vi "R1SBRControl.vi"(8 "error constant":errorcluster, 11 "LabVIEW Web Service":refnum<class "Web Service.lvclass">) -> (0 "error out":errorcluster)   [LabVIEW 2016]
uses:
  <vilib>/wsapi/Web Service.lvclass
  R1Controls/R1SBR_SetParams.ctl
  <vilib>/Utility/Variable/NI_VariableUtilities.lvlib
panel:
  out "No phases":i32
  out "current time":timestamp
  out "Numeric":i32
  out "Numeric 2":i32
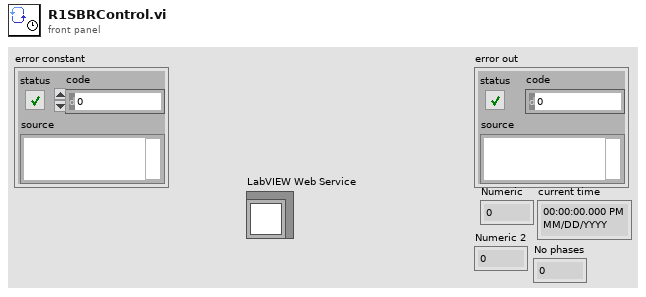
[diagram p1: front panel]
types:
  T1 = cluster{"Media Pump":bool, "Water Pump":bool, "Gas Pump":bool, "Effluent Pump":bool}
  T2 = typedef "R1SBR_SetParams.ctl" = cluster{"Phase":string, "Time, min":dbl, "SBR_Manual":cluster{"Media Pump":bool, "Water Pump":bool, "Gas Pump":bool, "Effluent Pump":bool}}[]
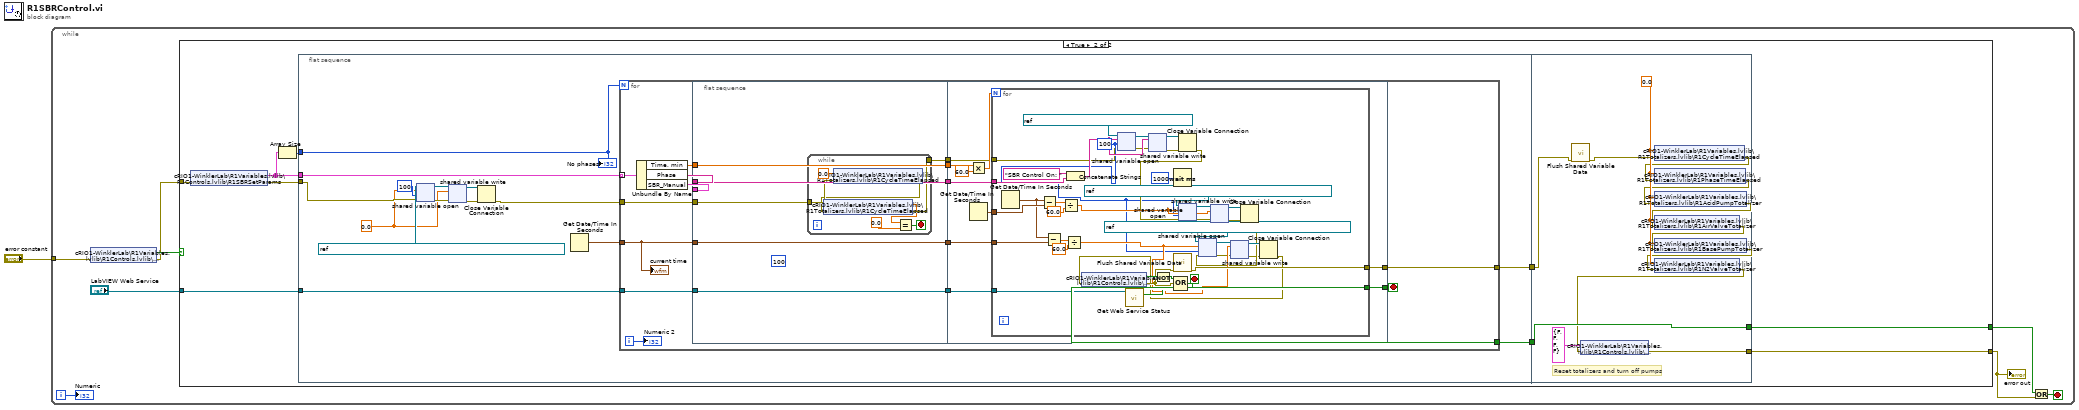
[diagram p0: block diagram]
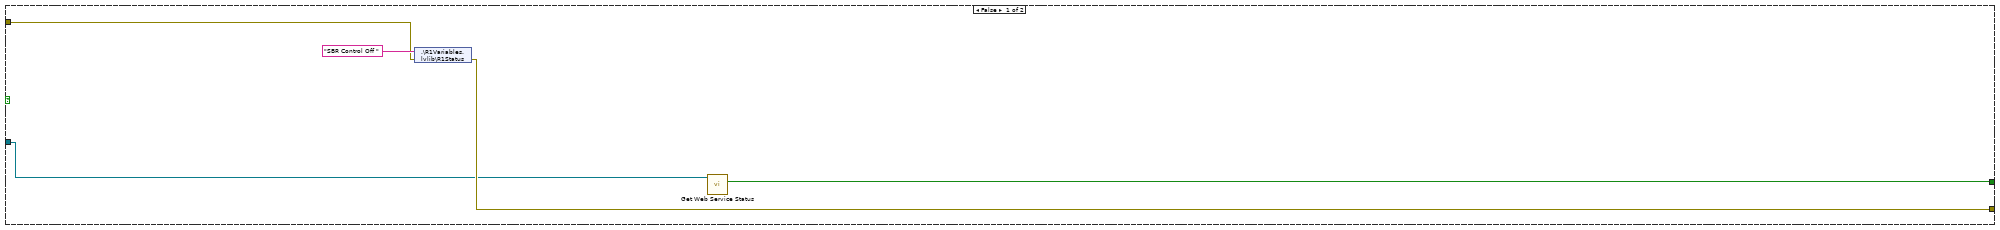
[diagram p2: hidden frame]
diagram:
  n1 = while {
    tunnel: "error constant" -> [w8]
    i -> [w2]
    stop <- w3 stop-if-true
    n2 = shared-variable "cRIO1-WinklerLab\\R1Variables.lvlib\\R1Controls.lvlib\\R1SBRSwitch"(error in=w8) -> (w9:bool, error out=w7:errorcluster)
    n3 = case shown="True" w9 {
      tunnel: "LabVIEW Web Service" -> [w11 w21]
      tunnel: w7 -> [w13 w20]
      tunnel: [w12 w17] -> w5
      tunnel: [w10 w15] -> w4
      frame False {
        n4 = shared-variable ".\\R1Variables.lvlib\\R1Status"("SBR Control Off " ("string"), error in=w13) -> (error out=w12:errorcluster)
        n5 = call <vilib>:"Get Web Service Status.vi"("LabVIEW Web Service"=w11) -> ("service stopping?"=w10:bool)  [unwired: 12 in, 2 out]
      }
      frame True {
        n6 = shared-variable "cRIO1-WinklerLab\\R1Variables.lvlib\\R1Controls.lvlib\\R1SBRSetParams"(error in=w20) -> (w22:T2, error out=w19:errorcluster)
        n7 = Array Size(array=w22) -> (size(s)=w23:i32)
        n8 = flat-sequence {
          tunnel: w22 -> [w37]
          tunnel: w23 -> [w38]
          tunnel: w21 -> [w36]
          tunnel: w19 -> [w26]
          tunnel: [w33] -> w18
          tunnel: [w35] -> w16
          tunnel: w18 -> [w119]
          tunnel: [w121] -> w17
          tunnel: [w120] -> w15
          tunnel: w16 -> [w120]
          frame #0 {
            w24 = 0.0 ("R1CycleTimeElapsed")
            n9 = shared-variable-open(refnum<k21> "ni.var.psp://crio1-winklerlab/R1Variables/R1Totalizers/R1CycleTimeElapsed" ("shared variable refnum in"), w26, w24, 100 ("timeout ms")) -> (w31:refnum<k21>, w29:errorcluster)  [unwired: 2 in]
            n10 = shared-variable-write(w31, w29, w24) -> (w30:refnum<k21>, w28:errorcluster)
            n11 = Close Variable Connection(8:w28, 11:w30) -> (0:w25:errorcluster)
            n12 = Get Date/Time In Seconds() -> (seconds since 1Jan1904=w34:timestamp)
            n13 = for {
              N: w38 -> [_]
              tunnel: w37 -> [w53] mode=indexing
              tunnel: w36 -> [w51]
              tunnel: w25 -> [w45]
              tunnel: [w43] -> w33
              tunnel: [w42] -> w35
              tunnel: w34 -> [w40]
              i -> [w41]
              stop <- w42 stop-if-true
              n14 = Unbundle By Name(w53) -> ("Time, min"=w48:dbl, "Phase"=w47:string, "SBR_Manual"=w52:T1)
              n15 = flat-sequence {
                tunnel: w48 -> [w58]
                tunnel: w52 -> [_]
                tunnel: w51 -> [w59]
                tunnel: [w59] -> w50
                tunnel: [w58] -> w49
                tunnel: w47 -> [w57]
                tunnel: [w57] -> w46
                tunnel: w45 -> [w54]
                tunnel: w40 -> [w56]
                tunnel: [w56] -> w44
                tunnel: [w55] -> w39
                tunnel: [w75] -> w42
                tunnel: w50 -> [w76]
                tunnel: w49 -> [w74]
                tunnel: w46 -> [w71]
                tunnel: w44 -> [w69]
                tunnel: [w68] -> w43
                tunnel: w39 -> [w67]
                frame #0 {
                  (unwired) 100 ("timeout ms")
                  n16 = while {
                    tunnel: w54 -> [w63]
                    tunnel: [w64] -> w55
                    stop <- w65 stop-if-true
                    n17 = shared-variable "cRIO1-WinklerLab\\R1Variables.lvlib\\R1Totalizers.lvlib\\R1CycleTimeElapsed"(0.0 ("R1CycleTimeElapsed"), error in=w63) -> (error out=w61:errorcluster)
                    n18 = shared-variable "cRIO1-WinklerLab\\R1Variables.lvlib\\R1Totalizers.lvlib\\R1CycleTimeElapsed"(error in=w61) -> (w60:dbl, error out=w64:errorcluster)
                    n19 = Equal?(x=w60, y=0.0 ("R1CycleTimeElapsed")) -> (x = y?=w65:bool)
                  }
                }
                frame #1 {
                  n20 = Get Date/Time In Seconds() -> (seconds since 1Jan1904=w70:timestamp)
                  n21 = Multiply(x=w74, y=60.0) -> (x*y=w72:dbl)
                  n22 = for {
                    N: w72 -> [_]
                    tunnel: w76 -> [w105]
                    tunnel: [w114] -> w75
                    tunnel: w71 -> [w112]
                    tunnel: w70 -> [w109]
                    tunnel: w69 -> [w106]
                    tunnel: [w100] -> w68
                    tunnel: w67 -> [w77]
                    stop <- w114 stop-if-true
                    w78 = 100 ("timeout ms")
                    n23 = Get Date/Time In Seconds() -> (seconds since 1Jan1904=w107:timestamp)
                    n24 = Subtract(x=w107, y=w109) -> (x-y=w110:dbl)
                    n25 = Subtract(x=w107, y=w106) -> (x-y=w103:dbl)
                    n26 = Divide(x=w110, y=60.0) -> (x/y=w86:dbl)
                    n27 = Divide(x=w103, y=60.0) -> (x/y=w95:dbl)
                    n28 = Concatenate Strings("SBR Control On: " ("string"), w112) -> (w82:string)
                    n29 = shared-variable-open(refnum<k21> "ni.var.psp://crio1-winklerlab/R1Variables/R1Status" ("shared variable refnum in"), w77, w82, w78) -> (w84:refnum<k21>, w81:errorcluster)  [unwired: 2 in]
                    n30 = call <vilib>:"Get Web Service Status.vi"("LabVIEW Web Service"=w105) -> ("service stopping?"=w104:bool)  [unwired: 12 in, 2 out]
                    n31 = shared-variable-write(w84, w81, w82) -> (w85:refnum<k21>, w80:errorcluster)
                    n32 = Wait (ms)(milliseconds to wait=u32 1000) -> ()  [unwired: 1 out]
                    n33 = Close Variable Connection(8:w80, 11:w85) -> (0:w79:errorcluster)
                    n34 = shared-variable-open(refnum<k21> "ni.var.psp://crio1-winklerlab/R1Variables/R1Totalizers/R1PhaseTimeElapsed" ("shared variable refnum in"), w79, w86, w78) -> (w93:refnum<k21>, w91:errorcluster)  [unwired: 2 in]
                    n35 = shared-variable-write(w93, w91, w86) -> (w94:refnum<k21>, w90:errorcluster)
                    n36 = Close Variable Connection(8:w90, 11:w94) -> (0:w89:errorcluster)
                    n37 = shared-variable-open(refnum<k21> "ni.var.psp://crio1-winklerlab/R1Variables/R1Totalizers/R1CycleTimeElapsed" ("shared variable refnum in"), w89, w95, w78) -> (w98:refnum<k21>, w88:errorcluster)  [unwired: 2 in]
                    n38 = shared-variable-write(w98, w88, w95) -> (w99:refnum<k21>, w87:errorcluster)
                    n39 = Close Variable Connection(8:w87, 11:w99) -> (0:w96:errorcluster)
                    n40 = shared-variable "cRIO1-WinklerLab\\R1Variables.lvlib\\R1Controls.lvlib\\R1SBRSwitch"(error in=w96) -> (w116:bool, error out=w101:errorcluster)
                    n41 = Not(x=w116) -> (.not. x?=w115:bool)
                    n42 = call <vilib>:"Flush Shared Variable Data.vi"("error in (no error)"=w101) -> ("error out"=w100:errorcluster)  [unwired: 10 in]
                    n43 = Compound Arithmetic op=OR(w115, w101, w104) -> (w114:bool)
                  }
                }
              }
              "Numeric 2" <- w41
              "current time" <- w40
            }
            "No phases" <- w38
          }
          frame #1 {
            w127 = 0.0 ("R1CycleTimeElapsed")
            # "Reset totalizers and turn off pumps"
            n44 = call <vilib>:"Flush Shared Variable Data.vi"("error in (no error)"=w119) -> ("error out"=w118:errorcluster)  [unwired: 10 in]
            n45 = shared-variable "cRIO1-WinklerLab\\R1Variables.lvlib\\R1Totalizers.lvlib\\R1CycleTimeElapsed"(w127, error in=w118) -> (error out=w126:errorcluster)
            n46 = shared-variable "cRIO1-WinklerLab\\R1Variables.lvlib\\R1Totalizers.lvlib\\R1PhaseTimeElapsed"(w127, error in=w126) -> (error out=w125:errorcluster)
            n47 = shared-variable "cRIO1-WinklerLab\\R1Variables.lvlib\\R1Totalizers.lvlib\\R1AcidPumpTotalizer"(w127, error in=w125) -> (error out=w124:errorcluster)
            n48 = shared-variable "cRIO1-WinklerLab\\R1Variables.lvlib\\R1Totalizers.lvlib\\R1AirValveTotalizer"(w127, error in=w124) -> (error out=w123:errorcluster)
            n49 = shared-variable "cRIO1-WinklerLab\\R1Variables.lvlib\\R1Totalizers.lvlib\\R1BasePumpTotalizer"(w127, error in=w123) -> (error out=w122:errorcluster)
            n50 = shared-variable "cRIO1-WinklerLab\\R1Variables.lvlib\\R1Totalizers.lvlib\\R1N2ValveTotalizer"(w127, error in=w122) -> (error out=w117:errorcluster)
            n51 = shared-variable "cRIO1-WinklerLab\\R1Variables.lvlib\\R1Controls.lvlib\\R1SBRManual"(T1 {"Media Pump"=FALSE, "Water Pump"=FALSE, "Gas Pump"=FALSE, "Effluent Pump"=FALSE} ("R1SBR_Manual"), error in=w117) -> (error out=w121:errorcluster)
          }
        }
      }
    }
    "error out" <- w5
    n52 = Or(x=w4, y=w5) -> (x .or. y?=w3:bool)
    "Numeric" <- w2
  }
